vi "IT8800-Configure Slew Rate.vi"(8 "error in":errorcluster, 10 "Slew Rate":dbl, 11 "IT8800 Setting In In":T1={"VISA Resource Name"="", "Baud Rate"=19200, "Stop Bits"=20, "Wait For Read(ms)"=0, "Interface Type"=enum."GPIB", "Limits"=[]} {"Stop Bits" items=["1.0"=10, "2.0"=20]; "Baud Rate" items=["2400"=2400, "4800"=4800, "9600"=9600, "19200"=19200]}) -> (0 "error out":errorcluster, 3 "IT8800 Setting In Out":T1={"VISA Resource Name"="", "Baud Rate"=19200, "Stop Bits"=20, "Wait For Read(ms)"=0, "Interface Type"=enum."GPIB", "Limits"=[]} {"Stop Bits" items=["1.0"=10, "2.0"=20]; "Baud Rate" items=["2400"=2400, "4800"=4800, "9600"=9600, "19200"=19200]})   [LabVIEW 2018]
uses:
  Data Def/IT8800-Setting.ctl
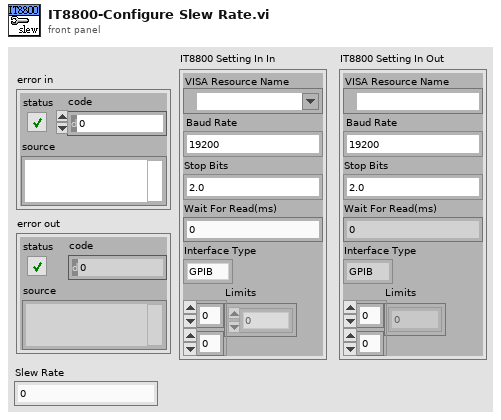
[diagram p1: front panel]
types:
  T1 = typedef "IT8800-Setting.ctl" = cluster{"VISA Resource Name":refnum<visa-resource-name>, "Baud Rate":u32, "Stop Bits":u16, "Wait For Read(ms)":u32, "Interface Type":enum16{"Unknow", "GPIB", "VXI", "GPIB-VXI", "Serial", "PXI", "TCPIP", "USB", "FireWire"}, "Limits":dbl[][]}
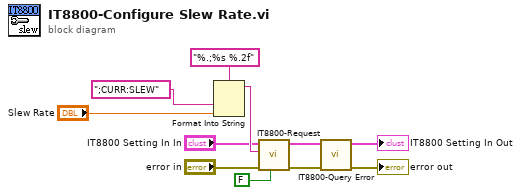
[diagram p0: block diagram]
diagram:
  n1 = Format Into String(format string="%.;%s %.2f", ";CURR:SLEW" ("input 1"), "Slew Rate") -> (resulting string=w11:string)  [unwired: 2 in, 1 out]
  n2 = call "IT8800-Request.vi"("Response?"=FALSE, "error in"="error in", "Command"=w11, "IT8800 Setting In In"="IT8800 Setting In In") -> ("error out"=w6:errorcluster, "IT8800 Setting In Out"=w5:T1)  [unwired: 5 in, 1 out]
  n3 = call "IT8800-Query Error.vi"("error in"=w6, "IT8800 Setting In In"=w5) -> ("error out"=→"error out":errorcluster, "IT8800 Setting In Out"=→"IT8800 Setting In Out":T1)  [unwired: 8 in]
